vi "Get Settings.vi"(8 "error in (no error)":errorcluster, 11 "DbgTimers in":refnum<class "DbgTimers.lvclass">) -> (0 "error out":errorcluster, 2 "Settings":T1, 3 "DbgTimers out":refnum<class "DbgTimers.lvclass">)   [LabVIEW 2017, in "DbgTimers.lvclass"]
doc: "Developed by Kevin Thompson\nkevin@thompsonengineering.net\n\nCopyright 2018-2020\nThompson Engineering, LLC"
uses:
  DbgTimers.lvclass
  DataTypes/Settings--cluster.ctl
  DbgTimers.lvclass/DbgTimers.ctl
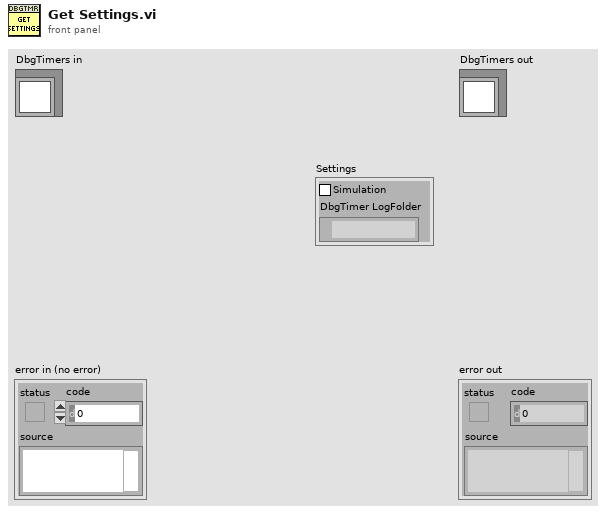
[diagram p1: front panel]
types:
  T1 = typedef "DbgTimers.lvclass/Settings--cluster.ctl" = cluster{"Simulation":bool, "DbgTimer LogFolder":path}
  T2 = typedef "DbgTimers.lvclass/ObjData--cluster.ctl" = cluster{"Settings":T1, "ReadData-placeholder":T3, "Timers":T4, "Enable msTick Logging":bool, "LogFile_msTickTimer":path}
  T3 = typedef "DbgTimers.lvclass/Read Data--cluster.ctl" = cluster{"Data":dbl}
  T4 = typedef "DbgTimers.lvclass/Timers--cluster.ctl" = cluster{"ms tick timers":T5[]}
  T5 = typedef "DbgTimers.lvclass/Millisecond Tick Timer--cluster.ctl" = cluster{"startTick":u32, "currentTick":u32, "elapsedTicks":u32, "totalElapsedTicks":u32}
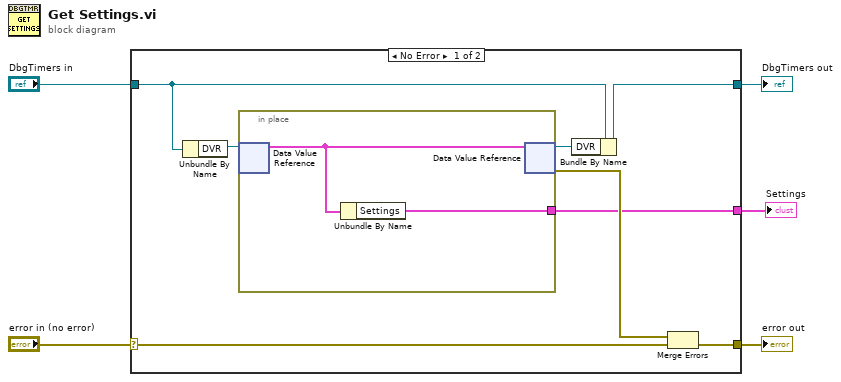
[diagram p0: block diagram]
diagram:
  n1 = case shown="No Error" "error in (no error)" {
    selector: "error in (no error)" -> [w13 w16]
    tunnel: [w8 w16] -> w4
    tunnel: [w9 w17] -> w2
    tunnel: "DbgTimers in" -> [w10 w17]
    tunnel: [w6 _] -> w1
    frame No Error {
      n2 = Unbundle By Name(w10) -> ("DVR"=w11:refnum<data-value>)
      n3 = in-place {
        in-place-border: [w14] -> w6
        n4 = in-place-dvr #1(w11) -> (w15:T2)  [unwired: 1 out]
        n5 = Unbundle By Name(w15) -> ("Settings"=w14:T1)
        n6 = in-place-dvr #1(w15) -> (w12:refnum<data-value>, w7:errorcluster)
      }
      n7 = Bundle By Name(cluster=w10, "DVR"=w12) -> (w9:refnum<class "DbgTimers.lvclass">)
      n8 = Merge Errors(w7, w13) -> (w8:errorcluster)
    }
    frame Error {
    }
  }
  "error out" <- w4
  "DbgTimers out" <- w2
  "Settings" <- w1
